vi "低层函数-event.vi"() -> ()   [LabVIEW 2018]
uses:
  <vilib>/userdefined/High Color/IMAQdx.ctl
  <vilib>/vision/Image Controls.llb/IMAQ Image.ctl
  <vilib>/vision/driver/IMAQdx.llb/IMAQdx Acquisition Mode.ctl
  <vilib>/vision/driver/IMAQdx.llb/IMAQdx Buffer Number Mode.ctl
  <vilib>/vision/driver/NI_Vision_Acquisition_Software.lvlib
  <resource>/objmgr/imaqdx.rc
panel:
  in  "布尔":bool
  out "Image Out":T1
  out "error out":errorcluster
  out "Image":T1(plugin-control)
  in  "error in":errorcluster
  in  "Session In":T2
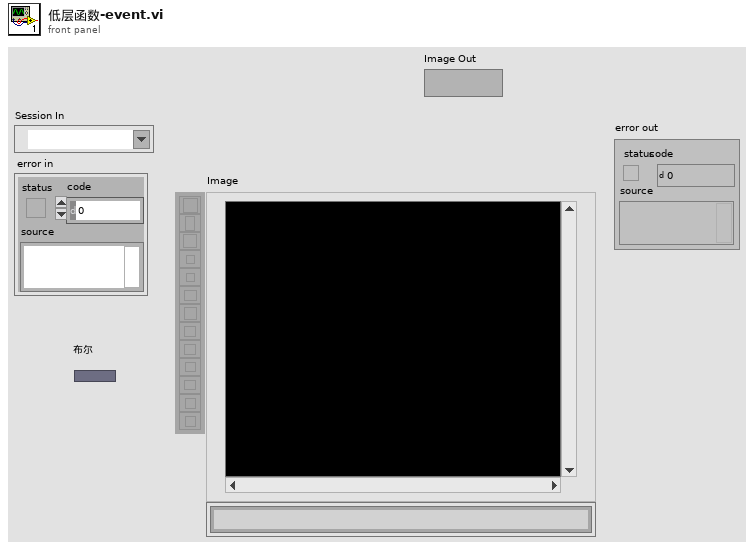
[diagram p1: front panel]
types:
  T1 = typedef "IMAQ Image.ctl" = refnum<image>
  T2 = typedef "IMAQdx.ctl" = refnum<k21>
  T3 = typedef "NI_Vision_Acquisition_Software.lvlib/IMAQdx Acquisition Mode.ctl" = enum32{"One Shot", "Continuous"}
  T4 = typedef "NI_Vision_Acquisition_Software.lvlib/IMAQdx Buffer Number Mode.ctl" = enum32{"Next", "Last", "Buffer Number", "Every", "Last New"}
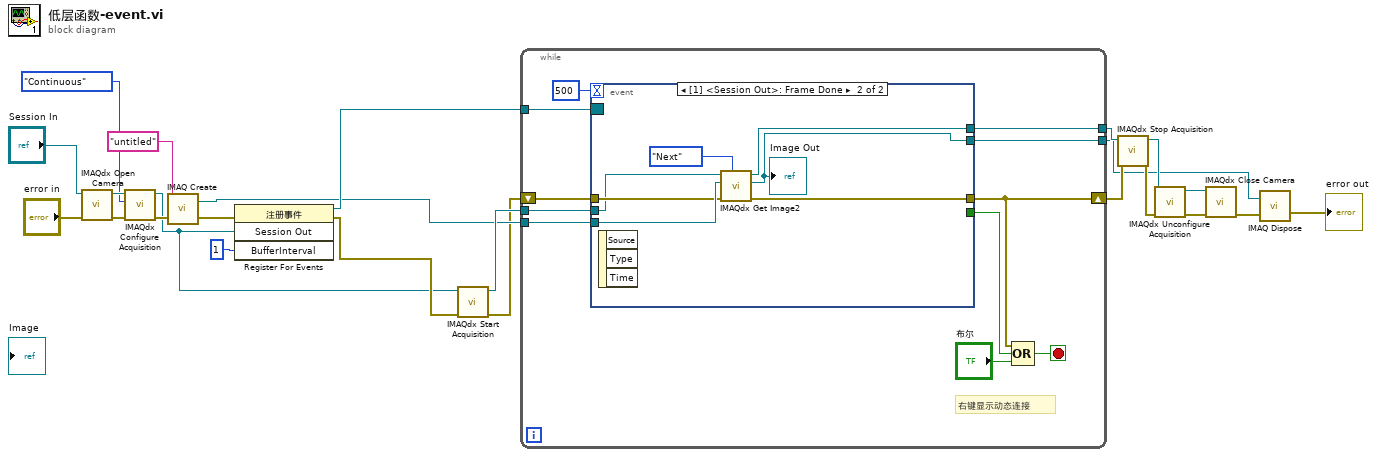
[diagram p0: block diagram]
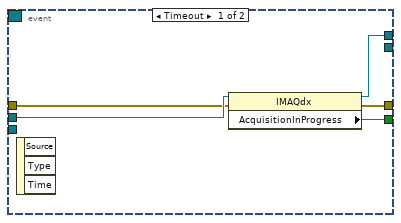
[diagram p2: hidden frame]
diagram:
  n1 = call <vilib>:"IMAQdx Open Camera.vi"("error in"="error in", "Session In"="Session In") -> ("error out"=w20:errorcluster, "Session Out"=w23:T2)  [unwired: 8 in]
  n2 = call <vilib>:"IMAQdx Configure Acquisition.vi"("error in"=w20, "Continuous?"=IMAQdx_Acquisition_Mode."Continuous", "Session In"=w23) -> ("error out"=w24:errorcluster, "Session Out"=w1:T2)  [unwired: 7 in]
  n3 = call "IMAQ Create"("Image Name"="untitled", "error in (no error)"=w24) -> ("New Image"=w9:T1, "error out"=w14:errorcluster)  [unwired: 3 in]
  n4 = register-events(error in=w14, w1, u32 1 ("BufferInterval")) -> (reference out=w12:refnum<event-registration>, error out=w10:errorcluster)  [unwired: 1 in]
  n5 = call <vilib>:"IMAQdx Start Acquisition.vi"("error in"=w10, "Session In"=w1) -> ("error out"=w4:errorcluster, "Session Out"=w11:T2)  [unwired: 8 in]
  n6 = while {
    tunnel: w12 -> [w35]
    tunnel: w9 -> [w33]
    tunnel: [w28] -> w7
    tunnel: w11 -> [w34]
    shift-right: [w29] -> w8
    shift-left: w4 -> [w26]
    tunnel: [w25] -> w3
    stop <- w30 stop-if-true
    # "右键显示动态连接"
    n7 = event shown="[1] <Session Out>: Frame Done" {
      selector: w35 -> [_ _]
      dyn-events: _ -> [_ _]
      timeout: 500 -> [_ _]
      tunnel: w34 -> [w40 w41]
      tunnel: w33 -> [_ w47]
      tunnel: [w37 w45] -> w29
      tunnel: [w39 w44] -> w28
      tunnel: [w38 _] -> w31
      tunnel: w26 -> [w36 w43]
      tunnel: [_ w42] -> w25
      event Timeout {
        n8 = event-data() -> ()  [unwired: 1 in, 3 out]
        n9 = property class="IMAQdx"(reference=w40, error in=w36) -> (reference out=w39:T2, error out=w37:errorcluster, "AcquisitionInProgress"=w38:bool)
      }
      event event #0x0 {
        n10 = event-data() -> ()  [unwired: 1 in, 3 out]
        n11 = call <vilib>:"IMAQdx Get Image2.vi"("Buffer Number Mode (Next)"=IMAQdx_Buffer_Number_Mode."Next", "error in"=w43, "Image In"=w47, "Session In"=w41) -> ("error out"=w45:errorcluster, "Image Out"=w42:T1, "Session Out"=w44:T2)  [unwired: 4 in, 1 out]
        "Image Out" <- w42
      }
    }
    n12 = Compound Arithmetic op=OR ("复合运算")(w29, w31, "布尔") -> (w30:bool)
  }
  n13 = call <vilib>:"IMAQdx Stop Acquisition.vi"("error in"=w8, "Session In"=w7) -> ("error out"=w6:errorcluster, "Session Out"=w5:T2)  [unwired: 8 in]
  n14 = call <vilib>:"IMAQdx Unconfigure Acquisition.vi"("error in"=w6, "Session In"=w5) -> ("error out"=w15:errorcluster, "Session Out"=w16:T2)  [unwired: 8 in]
  n15 = call <vilib>:"IMAQdx Close Camera.vi"("error in"=w15, "Session In"=w16) -> ("error out"=w18:errorcluster)  [unwired: 9 in]
  n16 = call "IMAQ Dispose"("Image"=w3, "error in (no error)"=w18) -> ("error out"=→"error out":errorcluster)  [unwired: 4 in]
